vi "ConsumeACKs(byID).vi"(8 "error in (no error)":errorcluster, 10 "ControlPacket in":refnum<class "ControlPacket.lvclass">, 11 "Session in":refnum<class "Session.lvclass">) -> (0 "error out":errorcluster, 1 "response prepared?":bool, 2 "ControlPacket response":refnum<class "ControlPacket.lvclass">, 3 "Session out":refnum<class "Session.lvclass">)   [LabVIEW 2013, in "MQTT Base.lvlib" / "Session.lvclass"]
uses:
  Session.lvclass
  <vilib>/LabVIEW Open Source Project/MQTT Control Packets/Control Packets/ControlPacket/ControlPacket.lvclass
  Session.lvclass/Session.ctl
  Pending ACKs -- cluster.ctl
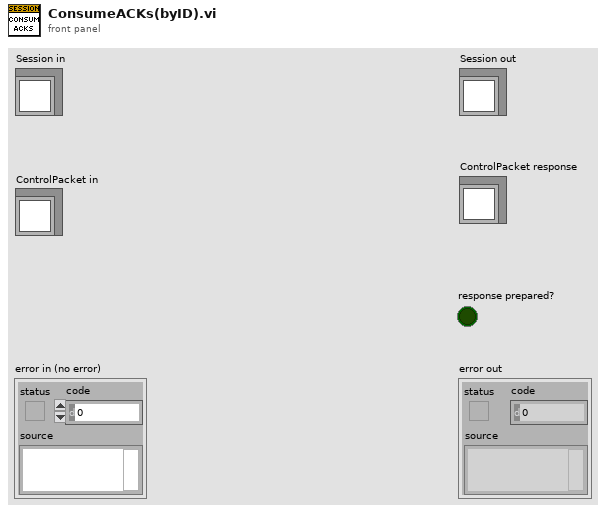
[diagram p1: front panel]
types:
  T1 = typedef "MQTT Base.lvlib/Session.lvclass/Pending ACKs -- cluster.ctl" = cluster{"Message":refnum<class "ControlPacket.lvclass">, "[ACK]":refnum<notifier>[], "Packet Identifier":u32}
  T2 = typedef "MQTT Base.lvlib/Session.lvclass/Session State -- cluster.ctl" = cluster{"CleanSession":bool, "Client ID":string, "Subscriptions":T3[], "Pending Transmissions":T5[], "Pending ACK map":variant}
  T3 = typedef "MQTT_Control_Packets.lvlib/SUBSCRIBE.lvclass/Topic Subscription -- cluster.ctl" = cluster{"Topic Filter":string, "QoS":T4}
  T4 = typedef "MQTT_Control_Packets.lvlib/ControlPacket.lvclass/QualityOfService -- enum.ctl" = enum16{"0 (At Most Once)", "1 (At Least Once)", "2 (Exactly Once)"}
  T5 = typedef "MQTT_Control_Packets.lvlib/ControlPacket.lvclass/Pending Transmission -- cluster.ctl" = cluster{"Message":refnum<class "ControlPacket.lvclass">, "QoS":T4, "Tx-Rx":bool}
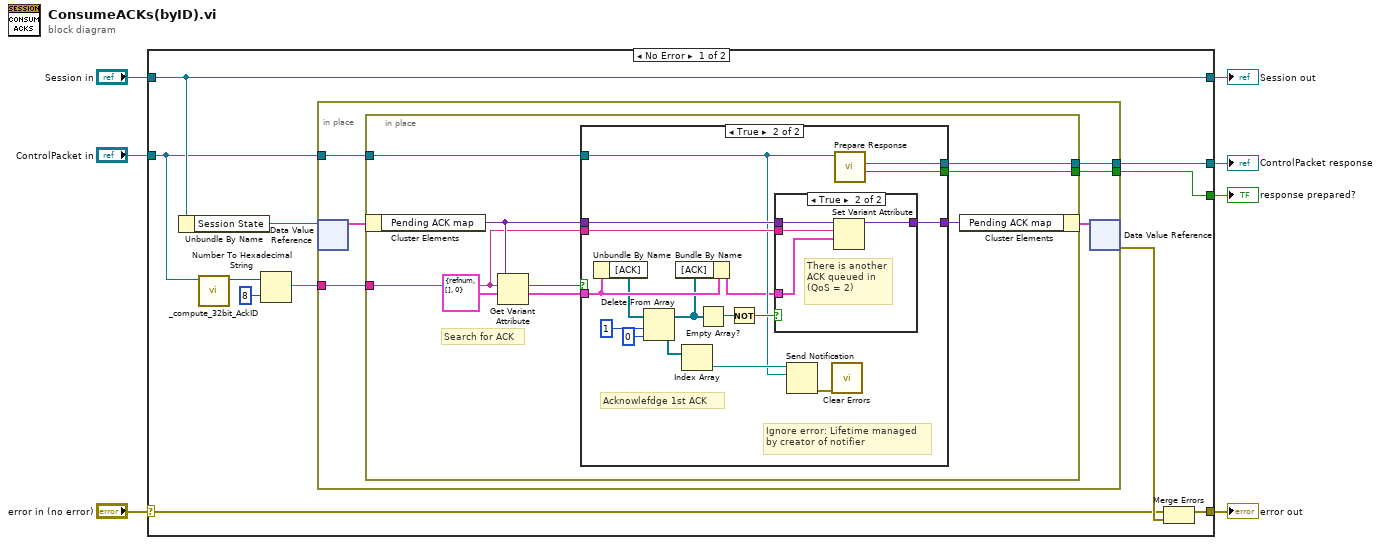
[diagram p0: block diagram]
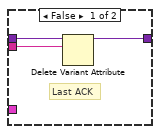
[diagram p3: hidden frame]
diagram:
  n1 = case shown="No Error" "error in (no error)" {
    selector: "error in (no error)" -> [w15 w59]
    tunnel: [w14 w59] -> w4
    tunnel: [w18 w60] -> w3
    tunnel: "Session in" -> [w18 w60]
    tunnel: "ControlPacket in" -> [w10 _]
    tunnel: [w9 _] -> w2
    tunnel: [w8 _] -> w1
    frame No Error {
      n2 = Unbundle By Name(w18) -> ("Session State"=w17:refnum<data-value>)
      n3 = call "_compute_32bit_AckID.vi"("ControlPacket in"=w10) -> ("ACK ID"=w13:u32)  [unwired: 10 in]
      n4 = Number To Hexadecimal String(1:i16 8 ("width (-)"), 2:w13) -> (0:w12:string)
      n5 = in-place {
        in-place-border: w12 -> [w22]
        in-place-border: w10 -> [w21]
        in-place-border: [w20] -> w9
        in-place-border: [w19] -> w8
        n6 = in-place-dvr #1(w17) -> (w24:T2)  [unwired: 1 out]
        n7 = in-place {
          in-place-border: w22 -> [w28]
          in-place-border: w21 -> [w27]
          in-place-border: [w26] -> w20
          in-place-border: [w25] -> w19
          # "Search for ACK"
          n8 = in-place-cluster #2(w24) -> ("Pending ACK map"=w30:variant)
          n9 = Get Variant Attribute(Variant=w30, name=w28, default value (empty Variant)=T1 {"Message"=refnum, "[ACK]"=[], "Packet Identifier"=0} ("Pending ACK")) -> (found=w32:bool, value=w29:T1)  [unwired: 1 in, 2 out]
          n10 = case shown="True" w32 {
            tunnel: w29 -> [_ w50]
            tunnel: [w34 w47] -> w31
            tunnel: w30 -> [w34 w48]
            tunnel: w28 -> [_ w46]
            tunnel: w27 -> [_ w36]
            tunnel: [_ w38] -> w26
            tunnel: [_ w37] -> w25
            frame False {
              # "No ack, No response"
            }
            frame True {
              # "Ignore error: Lifetime managed\nby creator of notifier"
              # "Acknowlefdge 1st ACK"
              n11 = Unbundle By Name(w50) -> ("[ACK]"=w44:refnum<notifier>[])
              n12 = Delete From Array(array=w44, length=1 ("index"), index=0) -> (deleted portion=w41:refnum<notifier>[], array with subset deleted=w43:refnum<notifier>[])
              n13 = Bundle By Name(cluster=w50, "[ACK]"=w43) -> (w35:T1)
              n14 = Index Array(array=w41) -> (element=w39:refnum<notifier>)  [unwired: 1 in]
              n15 = Empty Array?(array=w43) -> (empty?=w51:bool)
              n16 = Not(x=w51) -> (.not. x?=w49:bool)
              n17 = case shown="True" w49 {
                tunnel: w48 -> [w54 w58]
                tunnel: [w52 w57] -> w47
                tunnel: w46 -> [w53 w56]
                tunnel: w35 -> [_ w55]
                frame False {
                  # "Last ACK"
                  n18 = Delete Variant Attribute(6:w53, 7:w54) -> (3:w52:variant)  [unwired: 1 in, 2 out]
                }
                frame True {
                  # "There is another\nACK queued in\n(QoS = 2)"
                  n19 = Set Variant Attribute(Variant=w58, name=w56, value=w55) -> (Variant out=w57:variant)  [unwired: 1 in, 2 out]
                }
              }
              n20 = Send Notification(notification=w36, notifier=w39) -> (error out=w40:errorcluster)  [unwired: 1 in, 1 out]
              n21 = call <vilib>:"Clear Errors.vi"("error in (no error)"=w40) -> ()  [unwired: 6 in, 1 out]
              n22 = call-dynamic "Prepare Response.vi"("ControlPacket in"=w36) -> ("response prepared?"=w37:bool, "ControlPacket response"=w38:refnum<class "ControlPacket.lvclass">)  [unwired: 7 in, 2 out]
            }
          }
          n23 = in-place-cluster #2("Pending ACK map"=w31) -> (w23:T2)
        }
        n24 = in-place-dvr #1(w23) -> (w16:errorcluster)  [unwired: 1 out]
      }
      n25 = Merge Errors(w15, w16) -> (w14:errorcluster)
    }
    frame Error {
    }
  }
  "error out" <- w4
  "Session out" <- w3
  "response prepared?" <- w1
  "ControlPacket response" <- w2
